vi "SaveResultToMES.vi"(0 "class data in":refnum<class "CMESAPI.lvclass">, 5 "serialNumber":string, 7 "equipment":string, 11 "error in (no error)":errorcluster) -> (4 "class data out":refnum<class "CMESAPI.lvclass">, 6 "Result":bool, 8 "Report":string, 15 "error out":errorcluster)   [LabVIEW 2020, in "Salcomp-MES.lvlib" / "CMESAPI.lvclass"]
uses:
  CMESAPI.lvclass
  CMESAPI.lvclass/CMESAPI.ctl
  E:/Git/Libraries/develop/CME-API/CMESAPI_Fw4.0_1.9.2/CMESAPI.dll
  CMESAPI_Fw4.0_1.9.2/CMESAPI.dll
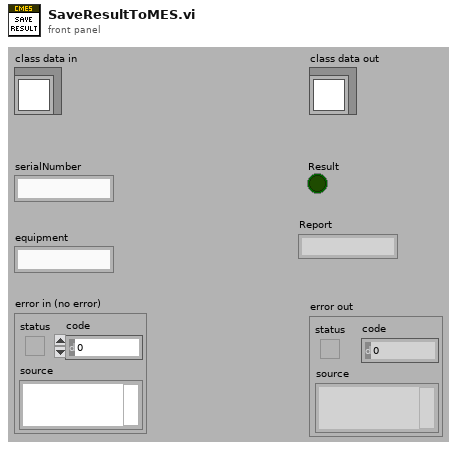
[diagram p1: front panel]
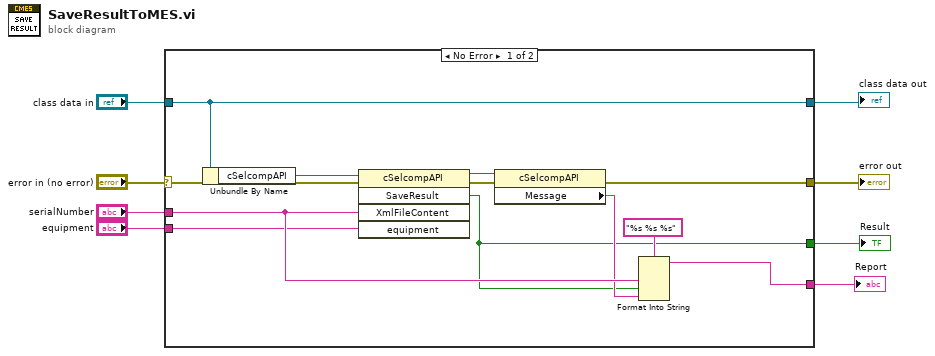
[diagram p0: block diagram]
diagram:
  n1 = case shown="No Error" "error in (no error)" {
    selector: "error in (no error)" -> [w18 w22]
    tunnel: [w15 w22] -> w7
    tunnel: "class data in" -> [w20 w21]
    tunnel: [w20 w21] -> w5
    tunnel: "serialNumber" -> [w13 _]
    tunnel: [w11 _] -> w2
    tunnel: "equipment" -> [w10 _]
    tunnel: [w9 _] -> w1
    frame No Error {
      n2 = Unbundle By Name(w20) -> ("cSelcompAPI"=w19:refnum<k24>)
      n3 = invoke on="Invoke Node" class="cSelcompAPI" method="SaveResult"(reference=w19, error in=w18, "XmlFileContent"=w13, "equipment"=w10) -> (reference out=w14:refnum<k24>, error out=w16:errorcluster, "SaveResult"=w11:bool)  [unwired: 1 in, 2 out]
      n4 = property class="cSelcompAPI"(reference=w14, error in=w16) -> (error out=w15:errorcluster, "Message"=w12:string)  [unwired: 1 out]
      n5 = Format Into String(format string="%s %s %s", w13, w11, w12) -> (resulting string=w9:string)  [unwired: 2 in, 1 out]
    }
    frame Error {
    }
  }
  "error out" <- w7
  "class data out" <- w5
  "Result" <- w2
  "Report" <- w1
